vi "DSF.Engine.Timing.Get Offset.vi"(11 "Timing in":refnum<class "DSF.Engine.Timing.lvclass">) -> (2 "Offset":u64, 3 "Timing out":refnum<class "DSF.Engine.Timing.lvclass">)   [LabVIEW 2017, in "DSF.Engine.lvlib" / "DSF.Engine.Timing.lvclass"]
uses:
  Engine/Classes/Timing/DSF.Engine.Timing.lvclass
  Engine/Classes/Timing/DSF.Engine.Timing.lvclass/DSF.Engine.Timing.ctl
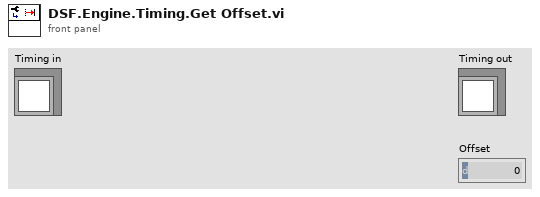
[diagram p1: front panel]
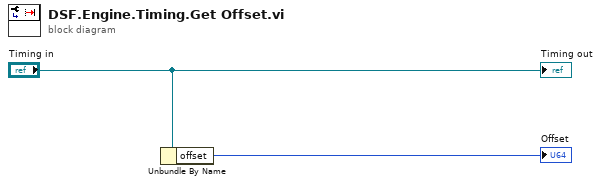
[diagram p0: block diagram]
diagram:
  n1 = Unbundle By Name("Timing in") -> ("offset"=→"Offset":u64)
  "Timing out" <- "Timing in"
